vi "4bar setpoint and immediate.vi"(6 "Operator X Button":bool, 7 "Hatch Setpoint":dbl, 8 "Operator Y Button":bool, 9 "Operator B Button":bool, 10 "Operator A Button":bool, 11 "Operator Right Joystick Y in":dbl) -> (3 "Output":T2 {"Control Mode" items=["PercentOutput"=0, "Position"=1, "Velocity"=2, "Current"=3, "Follower"=5, "MotionProfile"=6, "MotionMagic"=7, "MotionProfileArc"=10, "Disabled"=15]})   [LabVIEW 2018]
uses:
  <vilib>/Rock Robotics/WPI/ThirdParty/Phoenix-LabVIEW/Motor Controller/Controls/CTRE_Phoenix_MotorControl_ControlMode.ctl
  4barCommands.ctl
  Infrastructure/Constants.vi
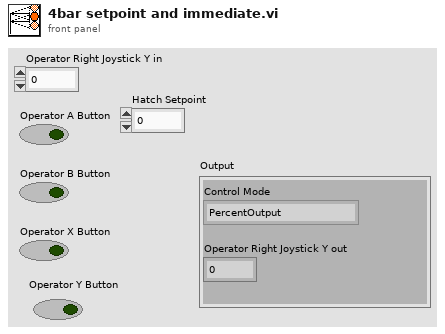
[diagram p1: front panel]
types:
  T1 = typedef "CTRE_Phoenix_MotorControl_ControlMode.ctl" = u16
  T2 = cluster{"Control Mode":T1, "Operator Right Joystick Y out":dbl}
  T3 = typedef "4barCommands.ctl" = enum16{"Immediate", "Hold", "Setpoint"}
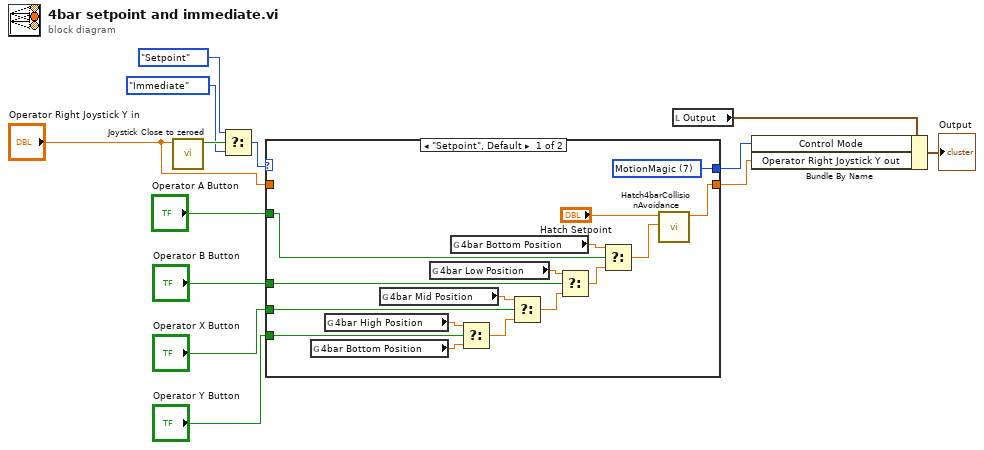
[diagram p0: block diagram]
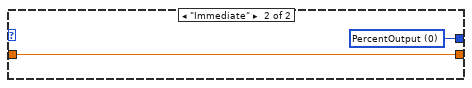
[diagram p2: hidden frame]
diagram:
  n1 = call "Joystick Close to zeroed.vi"("Joystick"="Operator Right Joystick Y in") -> ("=0?"=w12:bool)  [unwired: 10 in]
  n2 = Select(t=4barCommands."Setpoint", s=w12, f=4barCommands."Immediate") -> (s? t:f=w10:T3)
  n3 = case shown="\"Setpoint\", Default" w10 {
    tunnel: "Operator X Button" -> [w24 _]
    tunnel: "Operator B Button" -> [w23 _]
    tunnel: "Operator A Button" -> [w22 _]
    tunnel: "Operator Right Joystick Y in" -> [_ w31]
    tunnel: [w21 w30] -> w4
    tunnel: [w14 w31] -> w3
    tunnel: "Operator Y Button" -> [w19 _]
    frame "Setpoint", Default {
      w21 = T1 7 items=["PercentOutput"=0, "Position"=1, "Velocity"=2, "Current"=3, "Follower"=5, "MotionProfile"=6, "MotionMagic"=7, "MotionProfileArc"=10, "Disabled"=15] ("Control Mode")
      n4 = global read "Constants.vi" "4bar Bottom Position"() -> (w18:dbl)
      n5 = global read "Constants.vi" "4bar High Position"() -> (w20:dbl)
      n6 = global read "Constants.vi" "4bar Mid Position"() -> (w27:dbl)
      n7 = global read "Constants.vi" "4bar Low Position"() -> (w26:dbl)
      n8 = global read "Constants.vi" "4bar Bottom Position"() -> (w25:dbl)
      n9 = Select(t=w20, s=w19, f=w18) -> (s? t:f=w17:dbl)
      n10 = Select(t=w27, s=w24, f=w17) -> (s? t:f=w28:dbl)
      n11 = Select(t=w26, s=w23, f=w28) -> (s? t:f=w29:dbl)
      n12 = Select(t=w25, s=w22, f=w29) -> (s? t:f=w15:dbl)
      n13 = call "Hatch4barCollisionAvoidance.vi"("Current4barSetpoint"=w15, "Hatch Setpoint"="Hatch Setpoint") -> ("Modified 4bar setpoint"=w14:dbl)  [unwired: 9 in]
    }
    frame "Immediate" {
      w30 = T1 0 items=["PercentOutput"=0, "Position"=1, "Velocity"=2, "Current"=3, "Follower"=5, "MotionProfile"=6, "MotionMagic"=7, "MotionProfileArc"=10, "Disabled"=15] ("Control Mode")
    }
  }
  n14 = local read "Output"() -> (w1:T2)
  n15 = Bundle By Name(cluster=w1, "Control Mode"=w4, "Operator Right Joystick Y out"=w3) -> (→"Output":T2)
